vi "Control-Fuel.vi"(8 "Error In":errorcluster, 11 "DSI Reference":refnum<class "DCM-DSI.lvclass">) -> (0 "Error Out":errorcluster, 3 "DSI Reference":refnum<class "DCM-DSI.lvclass">)   [LabVIEW 2016, in "DSI-RT.lvlib"]
uses:
  DSI-RT.lvlib
  Classes/DCM-DSI/DCM-DSI.lvclass
  Shared/Typedefs/Engine-Channel.ctl
  <vilib>/addons/Software Calibration Management/xSCM/Controls/TBL2D.ctl
  Classes/DCM-DSI/Read Channels.vi
  Classes/DCM-DSI/Read EPTx Data.vi
  Classes/DCM-DSI/Write Channels.vi
  <vilib>/addons/Software Calibration Management/xSCM/CalPoint.xnode
  <vilib>/addons/Software Calibration Management/xSCM/Controls/TLU2D.ctl
  <vilib>/addons/Software Calibration Management/xSCM/FaultPoint.xnode
  <vilib>/addons/Software Calibration Management/xSCM/SCM-API.lvlib
  <vilib>/addons/Software Calibration Management/xSCM/ni_scm.dll
  Shared/DSI-Shared.lvlib
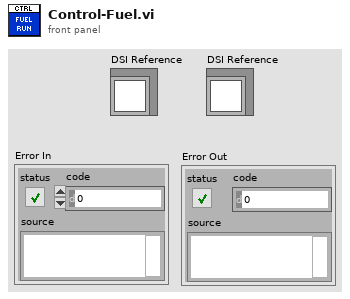
[diagram p1: front panel]
types:
  T1 = typedef "SCM-API.lvlib/TBL2D.ctl" = cluster{"X":sgl[], "Y":sgl[], "Z":sgl[][]}
  T2 = typedef "DSI-Shared.lvlib/Engine-Channel.ctl" = cluster{"Name":string, "Unit":string, "Value":sgl}
  T3 = typedef "DCM-DSI.lvclass/Channel.ctl" = cluster{"Name":string, "Unit":string, "Value":sgl}
  T4 = typedef "EPTx - RevA - RT.lvlib/EPTxData.ctl" = cluster{"Sync":bool, "CurrentCAD":sgl, "Speed [RPM]":sgl, "Config":bool, "Rcvg Primary":bool, "Stall":bool, "Overflow":bool, "Ratio Error":bool, "Pattern Error":bool, "Aux Warning":bool, "Watchdog Error":bool}
  T5 = typedef "SCM-API.lvlib/TLU2D.ctl" = cluster{"X":sgl, "Y":sgl, "Z":sgl}
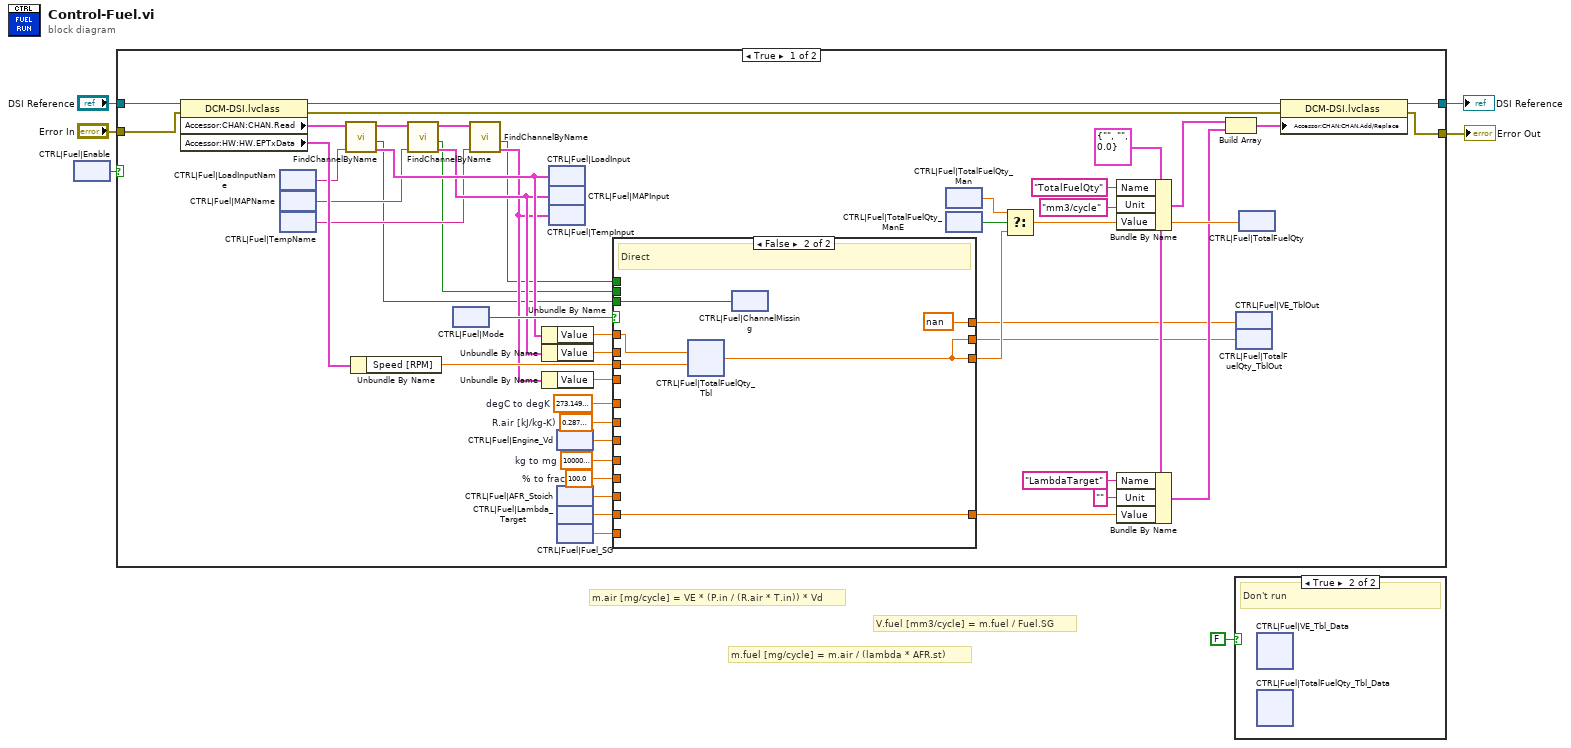
[diagram p0: block diagram]
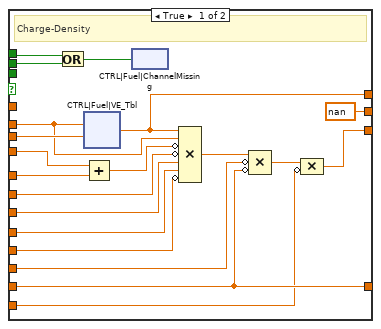
[diagram p3: hidden frame]
diagram:
  # "V.fuel [mm3/cycle] = m.fuel / Fuel.SG"
  # "m.fuel [mg/cycle] = m.air / (lambda * AFR.st)"
  # "m.air [mg/cycle] = VE * (P.in / (R.air * T.in)) * Vd"
  n1 = xnode "CTRL|Fuel|Enable"() -> ("Value"=w2:bool)
  n2 = case shown="True" w2 {
    tunnel: [w50 w261] -> w6
    tunnel: "Error In" -> [w49 w261]
    tunnel: "DSI Reference" -> [w48 w262]
    tunnel: [w47 w262] -> w3
    frame True {
      w21 = sgl 100.0  # % to frac
      w33 = sgl 1000000.0  # kg to mg
      w36 = sgl 273.15  # degC to degK
      w35 = sgl 0.287  # R.air [kJ/kg-K)
      w25 = T2 {"Name"="", "Unit"="", "Value"=0.0} ("element")
      n3 = property class="DCM-DSI.lvclass"(reference=w48, error in=w49) -> (reference out=w51:refnum<class "DCM-DSI.lvclass">, error out=w52:errorcluster, "Accessor:CHAN:CHAN.Read"=w19:T3[], "Accessor:HW:HW.EPTxData"=w53:T4)
      n4 = xnode "CTRL|Fuel|LoadInputName"() -> ("Value"=w16:string)
      n5 = xnode "CTRL|Fuel|MAPName"() -> ("Value"=w13:string)
      n6 = xnode "CTRL|Fuel|TempName"() -> ("Value"=w12:string)
      n7 = call "FindChannelByName.vi"("Name"=w16, "CTRL.Channels in"=w19) -> ("Channel"=w15:T2, "Searching"=w7:bool, "CTRL.Channels out"=w18:T2[])  [unwired: 6 in, 1 out]
      n8 = Unbundle By Name(w53) -> ("Speed [RPM]"=w44:sgl)
      n9 = call "FindChannelByName.vi"("Name"=w13, "CTRL.Channels in"=w18) -> ("Channel"=w14:T2, "Searching"=w8:bool, "CTRL.Channels out"=w17:T2[])  [unwired: 6 in, 1 out]
      n10 = xnode "CTRL|Fuel|Mode"() -> ("Value"=w37:bool)
      n11 = call "FindChannelByName.vi"("Name"=w12, "CTRL.Channels in"=w17) -> ("Channel"=w11:T2, "Searching"=w9:bool)  [unwired: 6 in, 2 out]
      n12 = Unbundle By Name(w15) -> ("Value"=w20:sgl)
      n13 = Unbundle By Name(w14) -> ("Value"=w39:sgl)
      n14 = Unbundle By Name(w11) -> ("Value"=w38:sgl)
      n15 = xnode "CTRL|Fuel|LoadInput"("Value"=w15) -> ()
      n16 = xnode "CTRL|Fuel|MAPInput"("Value"=w14) -> ()
      n17 = xnode "CTRL|Fuel|TempInput"("Value"=w11) -> ()
      n18 = xnode "CTRL|Fuel|Engine_Vd"() -> ("Value"=w34:sgl)
      n19 = xnode "CTRL|Fuel|AFR_Stoich"() -> ("Value"=w32:sgl)
      n20 = xnode "CTRL|Fuel|Lambda_Target"() -> ("Value"=w31:sgl)
      n21 = xnode "CTRL|Fuel|Fuel_SG"() -> ("Value"=w26:sgl)
      n22 = case shown="False" w37 {
        tunnel: w44 -> [w73 w113]
        tunnel: w39 -> [w72 _]
        tunnel: [w61 w111] -> w24
        tunnel: w38 -> [w70 _]
        tunnel: w36 -> [w69 _]
        tunnel: w35 -> [w68 _]
        tunnel: w34 -> [w67 _]
        tunnel: w33 -> [w66 _]
        tunnel: w32 -> [w65 _]
        tunnel: w31 -> [w64 w112]
        tunnel: [w64 w112] -> w28
        tunnel: w26 -> [w62 _]
        tunnel: [w59 sgl nan] -> w23
        tunnel: [sgl nan ("Z") w111] -> w22
        tunnel: w21 -> [w57 _]
        tunnel: w20 -> [_ w109]
        tunnel: w9 -> [w55 _]
        tunnel: w8 -> [w54 _]
        tunnel: w7 -> [_ w108]
        frame True {
          # "Charge-Density"
          n23 = Or(x=w55, y=w54) -> (x .or. y?=w56:bool)
          n24 = xnode "CTRL|Fuel|VE_Tbl"("Y Index"=w73, "X Index"=w72) -> ("Z"=w59:sgl)
          n25 = Add(x=w70, y=w69) -> (x+y=w71:sgl)
          n26 = xnode "CTRL|Fuel|ChannelMissing"("Fault"=w56) -> ()
          n27 = Compound Arithmetic op=MULTIPLY(w59, w72, invert w71, invert w68, w67, w66, invert w57) -> (w58:sgl)
          n28 = Compound Arithmetic op=MULTIPLY(w58, invert w65, invert w64) -> (w63:sgl)
          n29 = Compound Arithmetic op=MULTIPLY(w63, invert w62) -> (w61:sgl)
        }
        frame False {
          # "Direct"
          n30 = xnode "CTRL|Fuel|TotalFuelQty_Tbl"("Y Index"=w113, "X Index"=w109) -> ("Z"=w111:sgl)
          n31 = xnode "CTRL|Fuel|ChannelMissing"("Fault"=w108) -> ()
        }
      }
      n32 = xnode "CTRL|Fuel|TotalFuelQty_Man"() -> ("Value"=w45:sgl)
      n33 = xnode "CTRL|Fuel|TotalFuelQty_ManE"() -> ("Value"=w46:bool)
      n34 = Select(t=w45, s=w46, f=w24) -> (s? t:f=w40:sgl)
      n35 = Bundle By Name(cluster=w25, "Name"="TotalFuelQty", "Unit"="mm3/cycle", "Value"=w40) -> (w41:T2)
      n36 = Bundle By Name(cluster=w25, "Name"="LambdaTarget", "Unit"="", "Value"=w28) -> (w27:T2)
      n37 = Build Array(w41, w27) -> (w10:T2[])
      n38 = xnode "CTRL|Fuel|VE_TblOut"("Value"=w23) -> ()
      n39 = xnode "CTRL|Fuel|TotalFuelQty_TblOut"("Value"=w22) -> ()
      n40 = xnode "CTRL|Fuel|TotalFuelQty"("Value"=w40) -> ()
      n41 = property class="DCM-DSI.lvclass"(reference=w51, error in=w52, "Accessor:CHAN:CHAN.Add/Replace"=w10) -> (reference out=w47:refnum<class "DCM-DSI.lvclass">, error out=w50:errorcluster)
    }
    frame False {
    }
  }
  "Error Out" <- w6
  "DSI Reference" <- w3
  n42 = case shown="True" FALSE {
    frame False {
    }
    frame True {
      # "Don't run"
      n43 = xnode "CTRL|Fuel|VE_Tbl_Data"() -> ()  [unwired: 1 out]
      n44 = xnode "CTRL|Fuel|TotalFuelQty_Tbl_Data"() -> ()  [unwired: 1 out]
    }
  }
